vi "MGI User List FG.vi"(11 "Create? (F:Destroy)":bool) -> (3 "# Top Level Users":i32)   [LabVIEW 2020, in "MGI Error Reporter Base.lvclass"]
doc: "This functional global maintains a list of top level VIs that have created the Error Handler. If Create? is True, then the current top level VI is added to this list. If Create? is False, then the current top level VI is removed from the list, as is every remaining top level VI that is no longer running. \n\nAuthored by Shawn Walpole\nsupport@mooregoodideas.com\nwww.mooregoodideas.com\n\nCopyright (c) 2013, Moore Good Ideas, Inc.\n\nAll rights reserved.\n\nRedistribution and use in source and binary forms, with or without modification, are permitted provided that the following conditions are met:\n\n * Redistributions of source code must retain the above copyright notice, this list of conditions and the following disclaimer.\n * Redistributions in binary form must reproduce the above copyright notice, this list of conditions and the following disclaimer in the documentation and/or other materials provided with the distribution.\n * Neither the name of Moore Good Ideas, Inc. nor the names of its contributors may be used to endorse or promote products derived from this software without specific prior written permission.\n\nTHIS SOFTWARE IS PROVIDED BY THE COPYRIGHT HOLDERS AND CONTRIBUTORS \"AS IS\" AND ANY EXPRESS OR IMPLIED WARRANTIES, INCLUDING, BUT NOT LIMITED TO, THE IMPLIED WARRANTIES OF MERCHANTABILITY AND FITNESS FOR A PARTICULAR PURPOSE ARE DISCLAIMED. IN NO EVENT SHALL THE COPYRIGHT OWNER OR CONTRIBUTORS BE LIABLE FOR ANY DIRECT, INDIRECT, INCIDENTAL, SPECIAL, EXEMPLARY, OR CONSEQUENTIAL DAMAGES (INCLUDING, BUT NOT LIMITED TO, PROCUREMENT OF SUBSTITUTE GOODS OR SERVICES; LOSS OF USE, DATA, OR PROFITS; OR BUSINESS INTERRUPTION) HOWEVER CAUSED AND ON ANY THEORY OF LIABILITY, WHETHER IN CONTRACT, STRICT LIABILITY, OR TORT (INCLUDING NEGLIGENCE OR OTHERWISE) ARISING IN ANY WAY OUT OF THE USE OF THIS SOFTWARE, EVEN IF ADVISED OF THE POSSIBILITY OF SUCH DAMAGE."
uses:
  <userlib>/_MGI/Error Reporter/MGI Error Reporter Base/MGI Error Reporter Base.lvclass
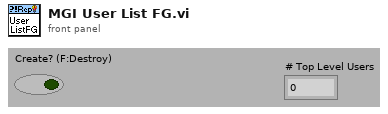
[diagram p1: front panel]
types:
  T1 = enum32{"Bad", "Idle", "Run top level", "Running"}[]
  T2 = enum32{"Bad", "Idle", "Run top level", "Running"}
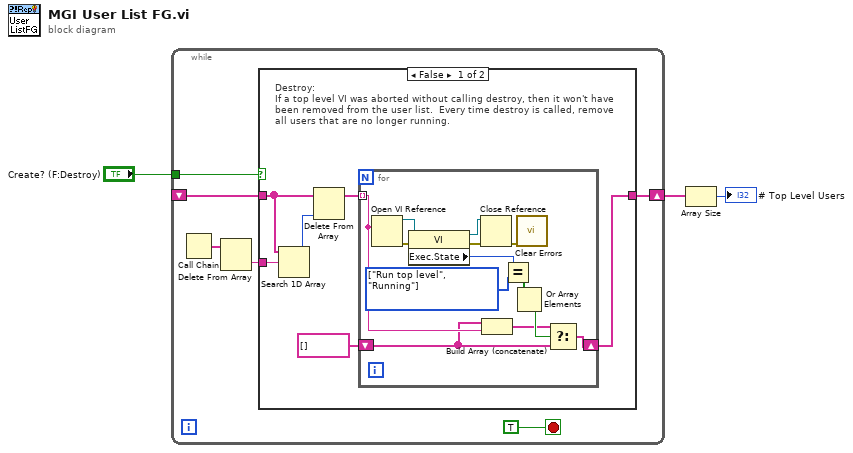
[diagram p0: block diagram]
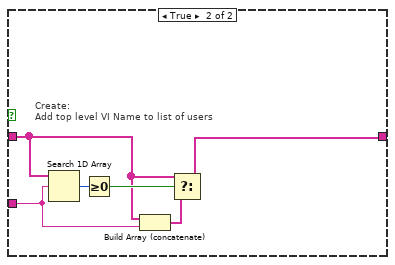
[diagram p2: hidden frame]
diagram:
  n1 = while {
    shift-right: [w7] -> w2
    shift-left: _ -> [w6]
    tunnel: "Create? (F:Destroy)" -> [w4]
    stop <- TRUE stop-if-true
    n2 = Call Chain() -> (call chain=w9:string[])
    n3 = Delete From Array(array=w9) -> (deleted portion=w8:string)  [unwired: 2 in, 1 out]
    n4 = case shown="False" w4 {
      tunnel: w8 -> [w15 w32]
      tunnel: [w10 w30] -> w7
      tunnel: w6 -> [w13 w29]
      frame False {
        # "Destroy:\nIf a top level VI was aborted without calling destroy, then it won't have been removed from the user list.  Every time destroy is called, remove all users that are no longer running."
        n5 = Search 1D Array(1D array=w13, element=w15) -> (index of element=w14:i32)  [unwired: 1 out]
        n6 = Delete From Array(array=w13, index=w14) -> (array with subset deleted=w12:string[])  [unwired: 1 in, 1 out]
        n7 = for {
          tunnel: w12 -> [w19] mode=indexing
          shift-right: [w17] -> w10
          shift-left: string[] [] -> [w16]
          w25 = T1 [enum."Run top level", enum."Running"] items=["Bad", "Idle", "Run top level", "Running"]
          n8 = Open VI Reference(vi path=w19) -> (vi reference=w27:refnum<vi>, error out=w28:errorcluster)  [unwired: 1 in, 4 out]
          n9 = property class="VI"(reference=w27, error in=w28) -> (reference out=w21:refnum<vi>, error out=w23:errorcluster, "Exec.State"=w26:T2)
          n10 = Close Reference(reference=w21, error in (no error)=w23) -> (error out=w22:errorcluster)
          n11 = Build Array (concatenate)(w16, w19) -> (w18:string[])
          n12 = Equal?(x=w26, y=w25) -> (x = y?=w24:bool[])
          n13 = Or Array Elements(Boolean array=w24) -> (logical OR=w20:bool)
          n14 = call <vilib>:"Clear Errors.vi"("error in (no error)"=w22) -> ()  [unwired: 1 in, 6 out]
          n15 = Select(t=w18, s=w20, f=w16) -> (s? t:f=w17:string[])
        }
      }
      frame True {
        # "Create:\nAdd top level VI Name to list of users"
        n16 = Search 1D Array(1D array=w29, element=w32) -> (index of element=w34:i32)  [unwired: 1 out]
        n17 = Greater Or Equal To 0?(x=w34) -> (x >= 0?=w33:bool)
        n18 = Build Array (concatenate)(w29, w32) -> (w31:string[])
        n19 = Select(t=w29, s=w33, f=w31) -> (s? t:f=w30:string[])
      }
    }
  }
  n20 = Array Size(array=w2) -> (size(s)=→"# Top Level Users":i32)
